vi "Agilent PWM Calibrate.vi"(7 "Agilent PWM":T2, 8 "error in (no error)":errorcluster, 10 "Normalize? (T)":T1=TRUE, 11 "VISA Resource Name":refnum<visa-resource-name>) -> (0 "error out":errorcluster {"code" format="%.0x"}, 2 "Normalized?":T1, 3 "dup VISA Resource Name":refnum<visa-resource-name>)   [LabVIEW 2011]
uses:
  TypeDefs/Agilent PWM Instrument Info.ctl
  PWM Normalization State.ctl
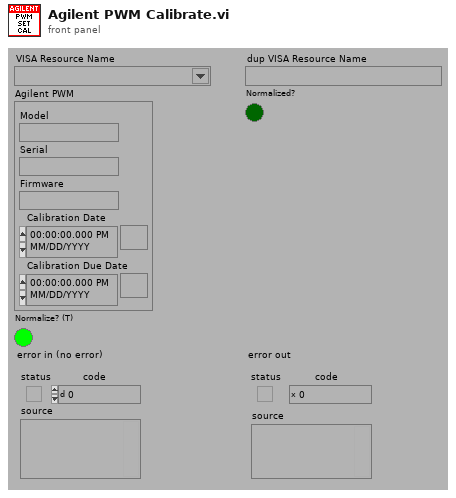
[diagram p1: front panel]
types:
  T1 = typedef "PWM Normalization State.ctl" = bool
  T2 = typedef "Agilent PWM Instrument Info.ctl" = cluster{"Model":string, "Serial":string, "Firmware":string, "Calibration Date":timestamp, "Calibration Due Date":timestamp}
  T3 = typedef "Agilent PWM Model.ctl" = enum16{"Not Supported", "E4418X", "E4419X", "U2000X"}
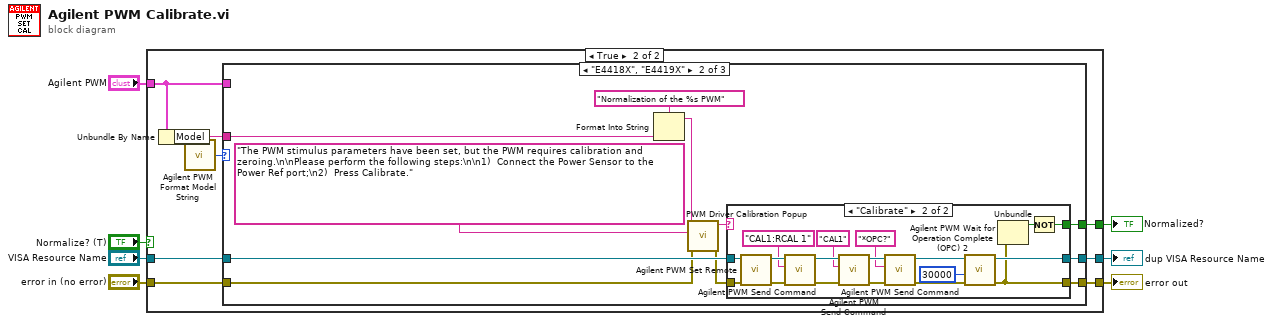
[diagram p0: block diagram]
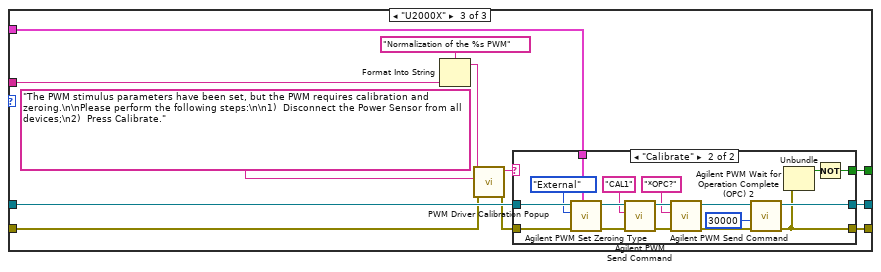
[diagram p5: hidden frame]
diagram:
  n1 = case shown="True" "Normalize? (T)" {
    tunnel: "Agilent PWM" -> [_ w10]
    tunnel: "VISA Resource Name" -> [w9 w17]
    tunnel: [w8 w16] -> w5
    tunnel: [w9 w15] -> w4
    tunnel: "error in (no error)" -> [w8 w14]
    tunnel: [_ w13] -> w1
    frame False {
    }
    frame True {
      n2 = Unbundle By Name(w10) -> ("Model"=w12:string)
      n3 = call "Agilent PWM Format Model String.vi"("Model"=w12) -> ("Model"=w11:T3)
      n4 = case shown="\"E4418X\", \"E4419X\"" w11 {
        tunnel: w17 -> [w19 w29 w61]
        tunnel: [w18 w28 w60] -> w16
        tunnel: [w19 w27 w59] -> w15
        tunnel: w14 -> [w18 w26 w58]
        tunnel: [_ w21 w53] -> w13
        tunnel: w12 -> [_ w20 w52]
        tunnel: w10 -> [_ _ w51]
        frame "Not Supported" {
        }
        frame "E4418X", "E4419X" {
          n5 = Format Into String(format string="Normalization of the %s PWM", w20) -> (resulting string=w24:string)  [unwired: 2 in, 1 out]
          n6 = call "PWM Driver Calibration Popup.vi"("error in (no error)"=w26, "Message"="The PWM stimulus parameters have been set, but the PWM requires calibration and zeroing.\n\nPlease perform the following steps:\n\n1)  Connect the Power Sensor to the Power Ref port;\n2)  Press Calibrate.", "Header"=w24) -> ("error out"=w25:errorcluster, "Dialog Response"=w22:string)  [unwired: 7 out]
          n7 = case shown="\"Calibrate\"" w22 {
            tunnel: w29 -> [w32 w50]
            tunnel: w25 -> [w31 w49]
            tunnel: [w31 w47] -> w28
            tunnel: [w32 w48] -> w27
            tunnel: [_ w45] -> w21
            frame Default {
            }
            frame "Calibrate" {
              n8 = call "Agilent PWM Set Remote.vi"("error in (no error)"=w49, "VISA Resource Name"=w50) -> ("error out"=w41:errorcluster, "dup VISA Resource Name"=w44:refnum<visa-resource-name>)  [unwired: 8 out]
              n9 = call "Agilent PWM Send Command.vi"("error in (no error)"=w41, "Command"="CAL1:RCAL 1" ("T button name (\"OK\")"), "VISA Resource Name"=w44) -> ("error out"=w42:errorcluster, "dup VISA Resource Name"=w43:refnum<visa-resource-name>)  [unwired: 3 in, 4 out]
              n10 = call "Agilent PWM Send Command.vi"("error in (no error)"=w42, "Command"="CAL1" ("T button name (\"OK\")"), "VISA Resource Name"=w43) -> ("error out"=w36:errorcluster, "dup VISA Resource Name"=w37:refnum<visa-resource-name>)  [unwired: 3 in, 4 out]
              n11 = call "Agilent PWM Send Command.vi"("error in (no error)"=w36, "Command"="*OPC?" ("T button name (\"OK\")"), "VISA Resource Name"=w37) -> ("error out"=w35:errorcluster, "dup VISA Resource Name"=w34:refnum<visa-resource-name>)  [unwired: 3 in, 4 out]
              n12 = call "Agilent PWM Wait for Operation Complete (OPC) 2.vi"("error in (no error)"=w35, "Timeout (300s)"=u32 30000, "VISA Resource Name"=w34) -> ("error out"=w47:errorcluster, "VISA Resource Name Out"=w48:refnum<visa-resource-name>)  [unwired: 6 in, 1 out]
              n13 = Unbundle(w47) -> ("status"=w46:bool)  [unwired: 2 out]
              n14 = Not(x=w46) -> (.not. x?=w45:bool)
            }
          }
        }
        frame "U2000X" {
          n15 = Format Into String(format string="Normalization of the %s PWM", w52) -> (resulting string=w56:string)  [unwired: 2 in, 1 out]
          n16 = call "PWM Driver Calibration Popup.vi"("error in (no error)"=w58, "Message"="The PWM stimulus parameters have been set, but the PWM requires calibration and zeroing.\n\nPlease perform the following steps:\n\n1)  Disconnect the Power Sensor from all devices;\n2)  Press Calibrate.", "Header"=w56) -> ("error out"=w57:errorcluster, "Dialog Response"=w54:string)  [unwired: 7 out]
          n17 = case shown="\"Calibrate\"" w54 {
            tunnel: w61 -> [w64 w68]
            tunnel: w57 -> [w63 w67]
            tunnel: [w63 w80] -> w60
            tunnel: [w64 w81] -> w59
            tunnel: [_ w78] -> w53
            tunnel: w51 -> [_ w65]
            frame Default {
            }
            frame "Calibrate" {
              n18 = call "Agilent PWM Set Zeroing Type.vi"("Agilent PWM"=w65, "error in (no error)"=w67, "Frequency (MHz)"=enum16{"Internal", "External"}."External", "VISA Resource Name"=w68) -> ("error out"=w76:errorcluster, "dup VISA Resource Name"=w77:refnum<visa-resource-name>)  [unwired: 6 in]
              n19 = call "Agilent PWM Send Command.vi"("error in (no error)"=w76, "Command"="CAL1" ("T button name (\"OK\")"), "VISA Resource Name"=w77) -> ("error out"=w72:errorcluster, "dup VISA Resource Name"=w73:refnum<visa-resource-name>)  [unwired: 3 in, 4 out]
              n20 = call "Agilent PWM Send Command.vi"("error in (no error)"=w72, "Command"="*OPC?" ("T button name (\"OK\")"), "VISA Resource Name"=w73) -> ("error out"=w71:errorcluster, "dup VISA Resource Name"=w70:refnum<visa-resource-name>)  [unwired: 3 in, 4 out]
              n21 = call "Agilent PWM Wait for Operation Complete (OPC) 2.vi"("error in (no error)"=w71, "Timeout (300s)"=u32 30000, "VISA Resource Name"=w70) -> ("error out"=w80:errorcluster, "VISA Resource Name Out"=w81:refnum<visa-resource-name>)  [unwired: 6 in, 1 out]
              n22 = Unbundle(w80) -> ("status"=w79:bool)  [unwired: 2 out]
              n23 = Not(x=w79) -> (.not. x?=w78:bool)
            }
          }
        }
      }
    }
  }
  "error out" <- w5
  "dup VISA Resource Name" <- w4
  "Normalized?" <- w1
